vi "StateToResults.vi"(7 "StateIn":T2 {"ILoad" format="%_6g"; "Fault Registers" format="%016x"; "VLoad" format="%_6g"; "VDCLink" format="%_6g"; "Detected Frequency" format="%1_6g"}) -> (4 "Results":T1, 8 "StateOut":T2 {"ILoad" format="%_6g"; "Fault Registers" format="%016x"; "VLoad" format="%_6g"; "VDCLink" format="%_6g"; "Detected Frequency" format="%1_6g"})   [LabVIEW 2017, in "AppStateMachine runtime.lvclass"]
uses:
  AppStateMachine runtime.lvclass
  State.ctl
  StateId.ctl
  LED_Color.ctl
  result user data.ctl
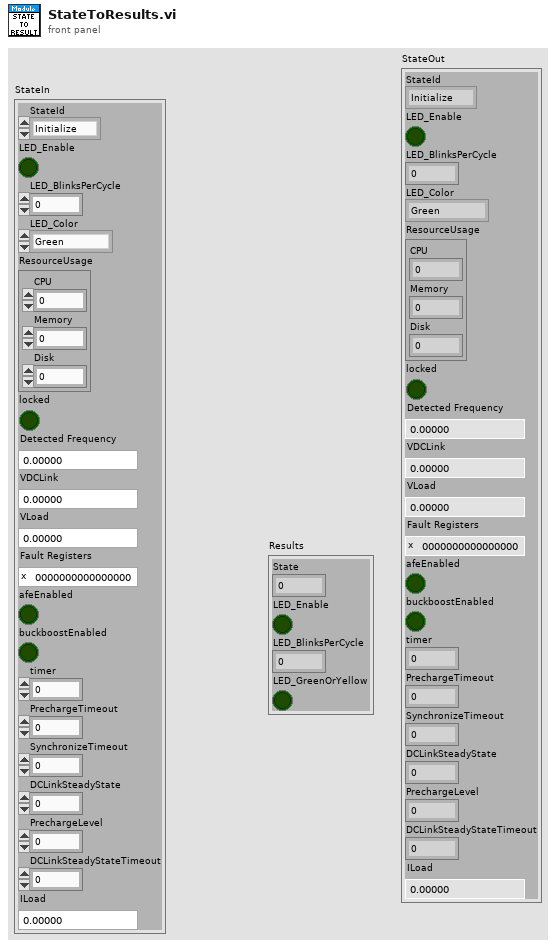
[diagram p1: front panel]
types:
  T1 = typedef "AppStateMachine runtime.lvclass/result user data.ctl" = cluster{"State":u16, "LED_Enable":bool, "LED_BlinksPerCycle":i32, "LED_GreenOrYellow":bool}
  T2 = typedef "AppStateMachine runtime.lvclass/State.ctl" = cluster{"StateId":T3, "LED_Enable":bool, "LED_BlinksPerCycle":i32, "LED_Color":T4, "ResourceUsage":cluster{"CPU":dbl, "Memory":dbl, "Disk":dbl}, "locked":bool, "Detected Frequency":dbl, "VDCLink":dbl, "VLoad":dbl, "Fault Registers":u64, "afeEnabled":bool, "buckboostEnabled":bool, "timer":u32, "PrechargeTimeout":u32, "SynchronizeTimeout":u32, "DCLinkSteadyState":dbl, "PrechargeLevel":dbl, "DCLinkSteadyStateTimeout":u32, "ILoad":dbl}
  T3 = typedef "AppStateMachine runtime.lvclass/StateId.ctl" = enum16{"Initialize", "Idle", "TunePLL", "TuneAFE", "TuneBuckBoost", "Precharge", "Synchronize", "Ready", "EnableAFE", "EnableBuckBoost", "Powered", "SafeState", "UnrecoverableSafeState"}
  T4 = typedef "AppStateMachine runtime.lvclass/LED_Color.ctl" = enum16{"Green", "Yellow"}
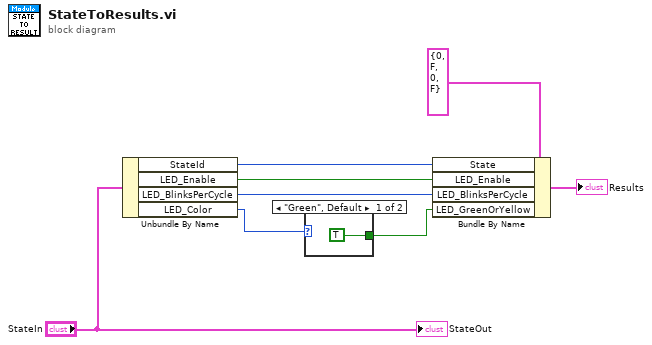
[diagram p0: block diagram]
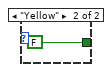
[diagram p2: hidden frame]
diagram:
  n1 = Unbundle By Name("StateIn") -> ("StateId"=w6:T3, "LED_Enable"=w4:bool, "LED_BlinksPerCycle"=w3:i32, "LED_Color"=w2:T4)
  n2 = case shown="\"Green\", Default" w2 {
    tunnel: [TRUE FALSE] -> w1
    frame "Green", Default {
    }
    frame "Yellow" {
    }
  }
  n3 = Bundle By Name(cluster=T1 {"State"=0, "LED_Enable"=FALSE, "LED_BlinksPerCycle"=0, "LED_GreenOrYellow"=FALSE} ("Results"), "State"=w6, "LED_Enable"=w4, "LED_BlinksPerCycle"=w3, "LED_GreenOrYellow"=w1) -> (→"Results":T1)
  "StateOut" <- "StateIn"
